vi "TTA_Issue_Command.vi"(8 "error in":errorcluster, 9 "Inputs":u16[](array[numeric]) format="%x", 10 "SubCommand":string(combo), 11 "MainCommand":string(combo)) -> (0 "error out":errorcluster)   [LabVIEW 2016]
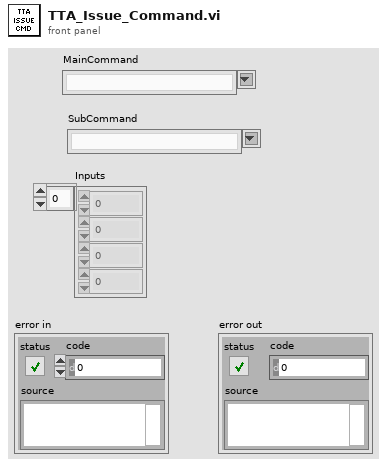
[diagram p1: front panel]
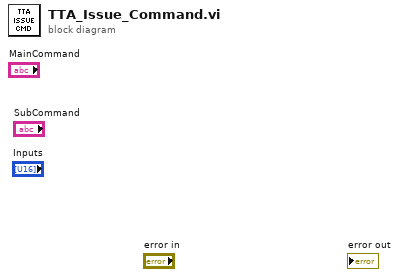
[diagram p0: block diagram]
diagram:
